vi "User Interface.vi"(8 "error in (no error)":errorcluster, 11 "User Interface in":refnum<class "User Interface.lvclass">) -> (0 "error out":errorcluster, 3 "User Interface out":refnum<class "User Interface.lvclass">)   [LabVIEW 2021, in "DSF Core.lvlib" / "Default Buffer Converter Transfers UI.lvclass"]
uses:
  Default Buffer Converter Transfers UI.lvclass
  Classes/User Interface/User Interface.lvclass
  Configurations/Default Buffer Converter Transfer Configuration.lvclass
  C:/dev/git/custom-devices/niveristand-data-sharing-framework-custom-device/Source/Core/Classes/Configuration/Configuration.lvclass
  Configurations/Default Buffer Converter Transfer Configuration.lvclass/Default Buffer Converter Transfer Configuration.ctl
panel:
  in  "Byte Order":u8(ring) items=["big-endian", "little-endian"]
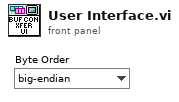
[diagram p1: front panel]
types:
  T1 = typedef "DSF Core.lvlib/Default Buffer Converter Transfer Configuration.lvclass/Transfer Configuration.ctl" = cluster{"byte order":T2}
  T2 = typedef "DSF Core.lvlib/DSF Byte Order.ctl" = enum8{"big-endian", "little-endian"}
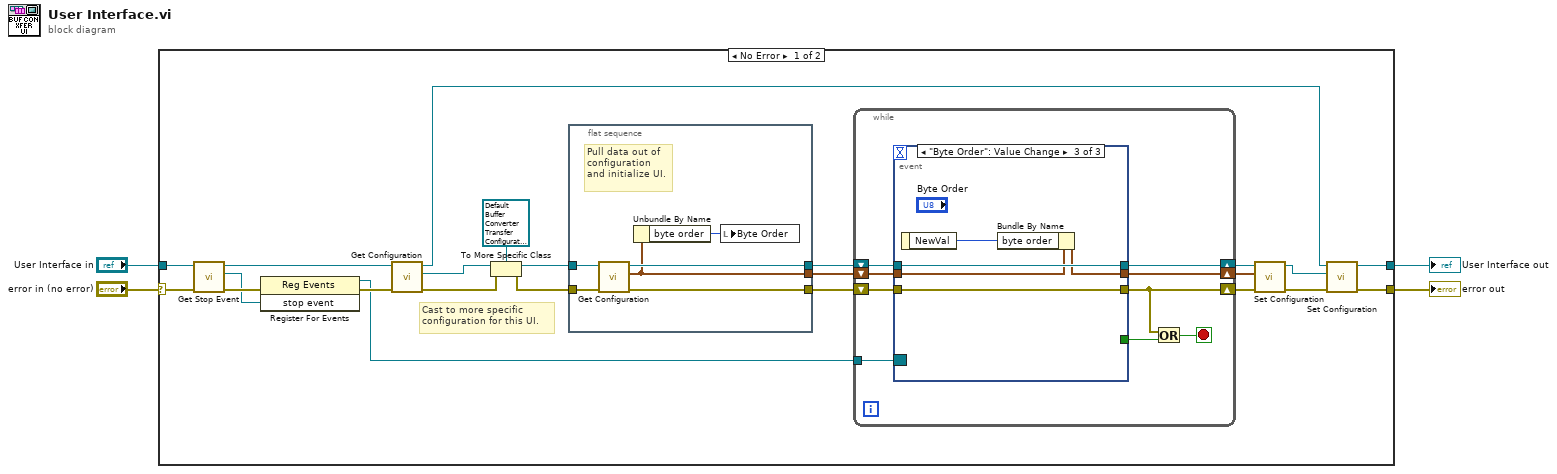
[diagram p0: block diagram]
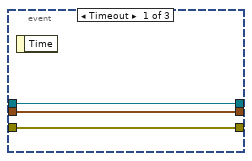
[diagram p2: hidden frame]
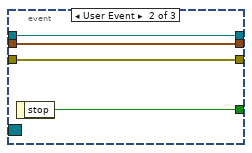
[diagram p3: hidden frame]
diagram:
  n1 = case shown="No Error" "error in (no error)" {
    selector: "error in (no error)" -> [w23 w56]
    tunnel: [w14 w56] -> w4
    tunnel: "User Interface in" -> [w22 w55]
    tunnel: [w13 w55] -> w1
    frame No Error {
      # "Cast to more specific configuration for this UI."
      n2 = call "Get Stop Event.vi"("error in (no error)"=w23, "User Interface in"=w22) -> ("error out"=w21:errorcluster, "stop event"=w20:refnum<user-event>, "User Interface out"=w19:refnum<class "User Interface.lvclass">)  [unwired: 7 in]
      n3 = register-events(error in=w21, w20) -> (reference out=w17:refnum<event-registration>, error out=w18:errorcluster)  [unwired: 1 in]
      n4 = call "Get Configuration.vi"("error in (no error)"=w18, "User Interface in"=w19) -> ("error out"=w16:errorcluster, "configuration"=w15:refnum<class "Configuration.lvclass">, "User Interface out"=w12:refnum<class "User Interface.lvclass">)  [unwired: 7 in]
      n5 = To More Specific Class(target class=refnum<class "Default Buffer Converter Transfer Configuration.lvclass"> refnum ("DSF Core.lvlib:DSF Buffer Converter Transfer Configuration.lvclass"), reference=w15, error in=w16) -> (specific class reference=w27:refnum<class "Default Buffer Converter Transfer Configuration.lvclass">, error out=w24:errorcluster)
      n6 = flat-sequence {
        tunnel: [w30] -> w25
        tunnel: w24 -> [w32]
        tunnel: w27 -> [w33]
        tunnel: [w31] -> w26
        tunnel: [w29] -> w10
        frame #0 {
          # "Pull data out of configuration and initialize UI."
          n7 = call "Get Configuration.vi"("error in (no error)"=w32, "DSF Buffer Converter Transfer Configuration in"=w33) -> ("error out"=w30:errorcluster, "configuration"=w29:T1, "DSF Buffer Converter Transfer Configuration out"=w31:refnum<class "Default Buffer Converter Transfer Configuration.lvclass">)  [unwired: 7 in]
          n8 = Unbundle By Name(w29) -> ("byte order"=w28:T2)
          n9 = local write "Byte Order"(w28) -> ()
        }
      }
      n10 = while {
        tunnel: w17 -> [w42]
        shift-right: [w40] -> w7
        shift-left: w25 -> [w41]
        shift-right: [w36] -> w9
        shift-left: w26 -> [w37]
        shift-right: [w34] -> w8
        shift-left: w10 -> [w35]
        stop <- w39 stop-if-true
        n11 = event shown="[2] \"Byte Order\": Value Change" {
          selector: w42 -> [_ _ _]
          dyn-events: _ -> [_ _ _]
          timeout: _ -> [_ _ _]
          tunnel: [_ w47 _] -> w38
          tunnel: w41 -> [w45 w49 w53]
          tunnel: [w45 w49 w53] -> w40
          tunnel: w37 -> [w44 w48 w54]
          tunnel: [w44 w48 w54] -> w36
          tunnel: w35 -> [w43 w46 w51]
          tunnel: [w43 w46 w52] -> w34
          event Timeout {
            n12 = event-data() -> ()  [unwired: 1 in, 1 out]
          }
          event User Event {
            n13 = event-data() -> ("stop"=w47:bool)  [unwired: 1 in]
          }
          event "Byte Order": Value Change {
            n14 = event-data() -> ("NewVal"=w50:u8)  [unwired: 1 in]
            n15 = Bundle By Name(cluster=w51, "byte order"=w50) -> (w52:T1)
          }
        }
        n16 = Or(x=w40, y=w38) -> (x .or. y?=w39:bool)
      }
      n17 = call "Set Configuration.vi"("error in (no error)"=w7, "configuration"=w8, "DSF Buffer Converter Transfer Configuration in"=w9) -> ("error out"=w5:errorcluster, "DSF Buffer Converter Transfer Configuration out"=w6:refnum<class "Default Buffer Converter Transfer Configuration.lvclass">)  [unwired: 7 in]
      n18 = call "Set Configuration.vi"("error in (no error)"=w5, "configuration"=w6, "User Interface in"=w12) -> ("error out"=w14:errorcluster, "User Interface out"=w13:refnum<class "User Interface.lvclass">)  [unwired: 7 in]
    }
    frame Error {
    }
  }
  "error out" <- w4
  "User Interface out" <- w1
